vi "D2SkillsTable - Public - Functions - Set Skill Levels.vi"(8 "error in (no error)":errorcluster, 10 "Levels":u8[](array[numeric]), 11 "D2SkillsTable in":refnum<class "D2SkillsTable.lvclass">) -> (0 "error out":errorcluster, 3 "D2SkillsTable out":refnum<class "D2SkillsTable.lvclass">)   [LabVIEW 2015, in "D2SkillsTable.lvclass"]
uses:
  D2SkillsTable.lvclass
  D2SkillsTable.lvclass/D2SkillsTable.ctl
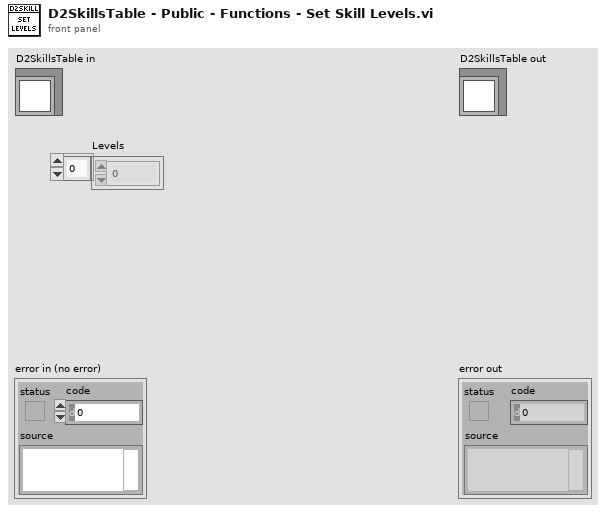
[diagram p1: front panel]
types:
  T1 = typedef "D2SkillsTable.lvclass/D2SkillsTable - Public - Controls - D2Skill.ctl" = cluster{"Skill Name":T2, "Offset":u8, "Level":u8}
  T2 = typedef "D2SkillsTable.lvclass/D2SkillsTable - Public - Controls - D2Skills.ctl" = u16
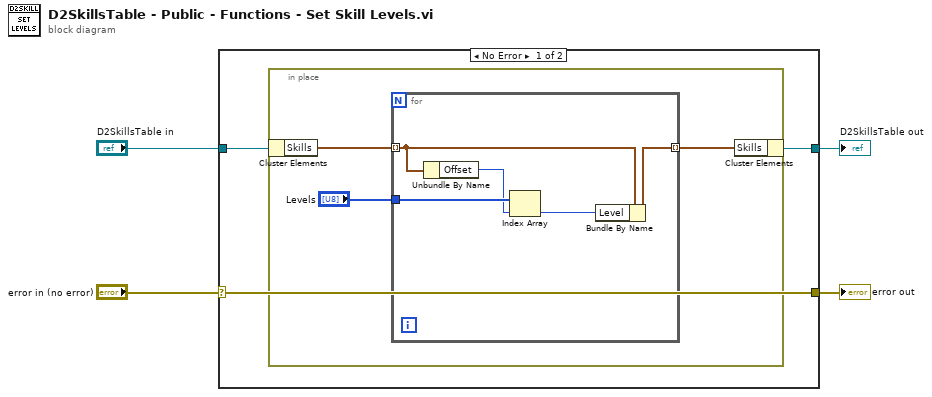
[diagram p0: block diagram]
diagram:
  n1 = case shown="No Error" "error in (no error)" {
    selector: "error in (no error)" -> [w5 w17]
    tunnel: [w5 w17] -> w3
    tunnel: [w6 w16] -> w1
    tunnel: "D2SkillsTable in" -> [w7 w16]
    frame No Error {
      n2 = in-place {
        n3 = in-place-cluster #1(w7) -> ("Skills"=w10:T1[])
        n4 = for {
          tunnel: w10 -> [w13] mode=indexing
          tunnel: "Levels" -> [w15]
          tunnel: [w12] -> w8 mode=indexing
          n5 = Unbundle By Name(w13) -> ("Offset"=w14:u8)
          n6 = Index Array(array=w15, index=w14) -> (element=w11:u8)
          n7 = Bundle By Name(cluster=w13, "Level"=w11) -> (w12:T1)
        }
        n8 = in-place-cluster #1("Skills"=w8) -> (w6:refnum<class "D2SkillsTable.lvclass">)
      }
    }
    frame Error {
    }
  }
  "error out" <- w3
  "D2SkillsTable out" <- w1
